vi "Image File Dialog.vi"(11 "Control Ref Queue":T2) -> ()   [LabVIEW 2020, in "3D Plot.lvclass"]
uses:
  <vilib>/Math Plots/3D Math Plots/3D Plot/3D Plot/3D Plot.lvclass
  <vilib>/Math Plots/3D Math Plots/3D Plot/Action String/3DMathPlot Ctrl Act Queue.ctl
  <vilib>/Math Plots/3D Math Plots/3D Plot/Action String/3DMathPlot Ctrl Act Cluster.ctl
  <vilib>/Math Plots/3D Math Plots/3D Plot/Action String/3DMathPlot State Class.ctl
panel:
  in  "Warning Message":string="File path is invalid."
  in  "Export":string="Export"
  in  "Save":string="Save"
  in  "Tab Control":enum32{"Appearance", "Input & Output"}(tab)
  in  "Help":bool
  in  "Cancel":bool
  in  "OK":bool
  in  "Path":path
  in  "To File":bool
  in  "To Clipboard":bool=TRUE
  in  "File Format":T1(radio)
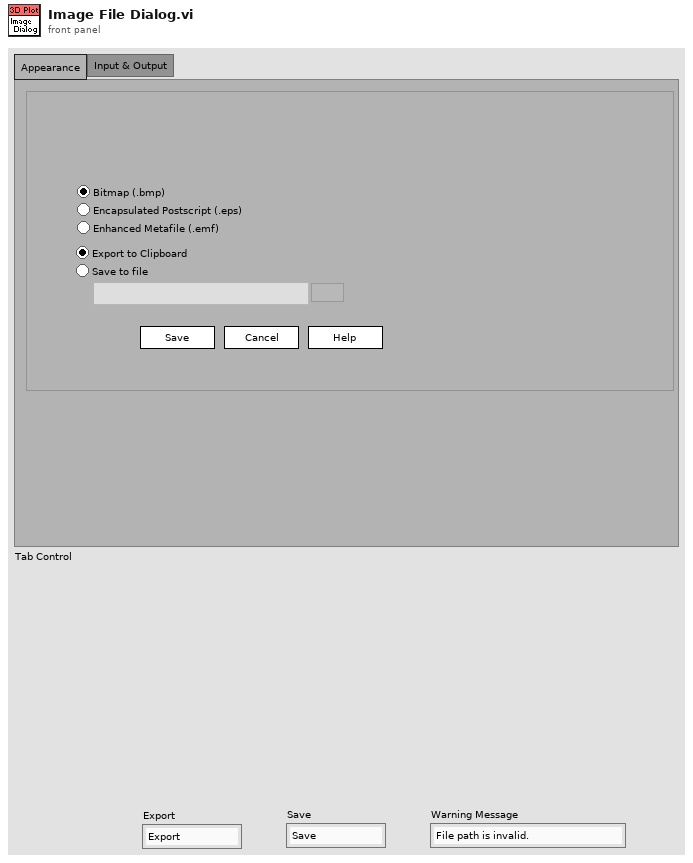
[diagram p1: front panel]
types:
  T1 = enum32{"Bitmap", "Postscript", "Metafile", "Mac PICT"}
  T2 = typedef "3DMathPlot Ctrl Act Queue.ctl" = refnum<queue>
  T3 = enum8{"Enabled", "Disabled", "Disabled and Grayed Out"}
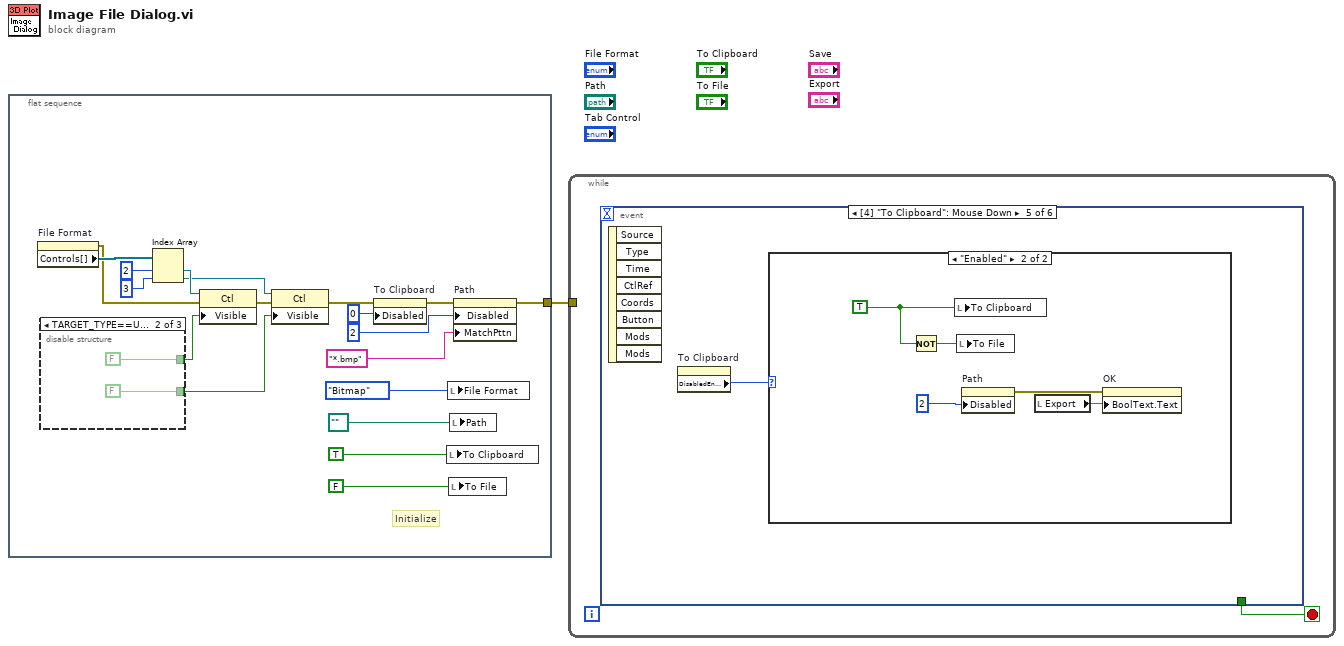
[diagram p0: block diagram]
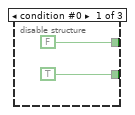
[diagram p2: hidden frame]
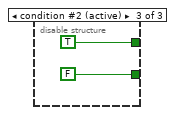
[diagram p3: hidden frame]
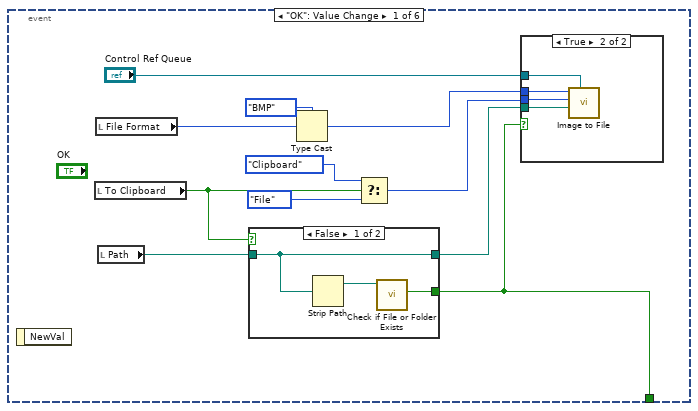
[diagram p4: hidden frame]
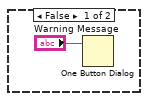
[diagram p5: hidden frame]
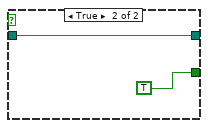
[diagram p6: hidden frame]
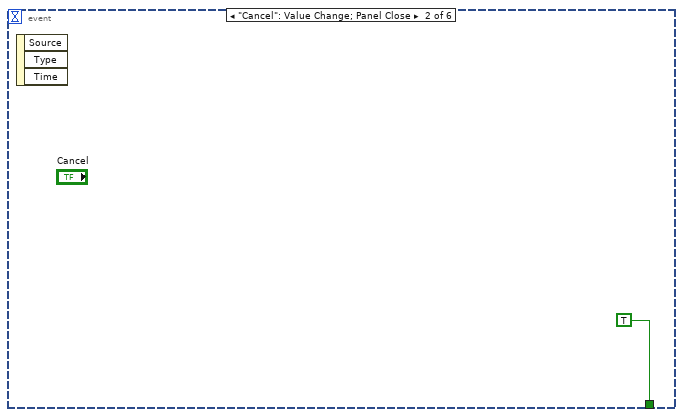
[diagram p7: hidden frame]
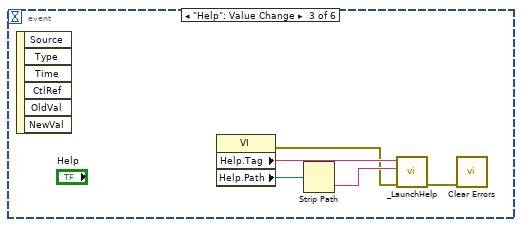
[diagram p8: hidden frame]
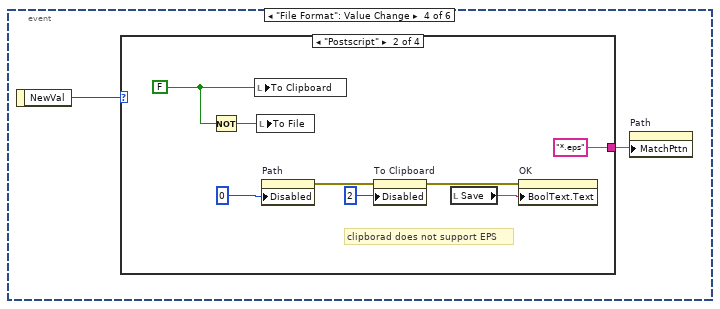
[diagram p9: hidden frame]
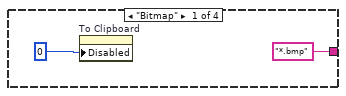
[diagram p10: hidden frame]
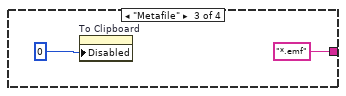
[diagram p11: hidden frame]
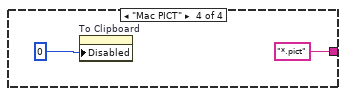
[diagram p12: hidden frame]
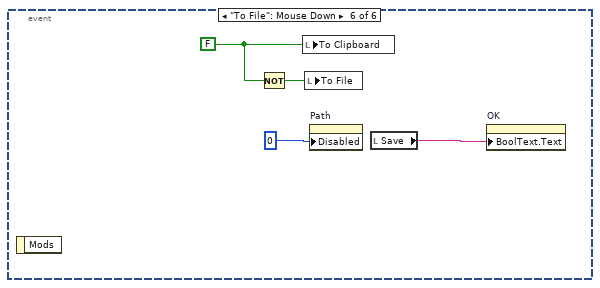
[diagram p14: hidden frame]
diagram:
  n1 = flat-sequence {
    tunnel: [w17] -> w1
    frame #0 {
      # "Initialize"
      n2 = property on="File Format" class="RadioBtnsControl (strict)"() -> (error out=w8:errorcluster, "Controls[]"=w11:refnum<vi>[])  [unwired: 2 in, 1 out]
      n3 = disable-structure shown="TARGET_TYPE==Unix" {
        disable-tunnel: [FALSE ("Visible") FALSE ("Visible") TRUE ("Visible")] -> w3
        disable-tunnel: [TRUE ("Visible") FALSE ("Visible") FALSE ("Visible")] -> w2
        frame condition #0 {
        }
        frame condition #1 {
        }
        frame condition #2 (active) {
        }
      }
      n4 = Index Array(array=w11, index #1=2 ("y"), index #2=3 ("y")) -> (element #1=w10:refnum<vi>, element #2=w6:refnum<vi>)
      n5 = property class="Ctl"(reference=w10, error in=w8, "Visible"=w3) -> (error out=w5:errorcluster)  [unwired: 1 out]
      n6 = property class="Ctl"(reference=w6, error in=w5, "Visible"=w2) -> (error out=w4:errorcluster)  [unwired: 1 out]
      n7 = property on="To Clipboard" class="Bool (strict)"(error in=w4, "Disabled"=u8 0) -> (error out=w16:errorcluster)  [unwired: 1 in, 1 out]
      n8 = local write "To Clipboard"(TRUE ("To Clipboard")) -> ()
      n9 = local write "File Format"(T1."Bitmap" ("File Format")) -> ()
      n10 = local write "To File"(FALSE ("To File")) -> ()
      n11 = local write "Path"(path "" ("Path")) -> ()
      n12 = property on="Path" class="Path"(error in=w16, "Disabled"=u8 2, "MatchPttn"="*.bmp" ("Browse Options:Match Pattern")) -> (error out=w17:errorcluster)  [unwired: 1 in, 1 out]
    }
  }
  n13 = while {
    tunnel: w1 -> [_]
    stop <- w27 stop-if-true
    n14 = event shown="[4] \"To Clipboard\": Mouse Down" {
      selector: _ -> [_ _ _ _ _ _]
      dyn-events: _ -> [_ _ _ _ _ _]
      timeout: _ -> [_ _ _ _ _ _]
      tunnel: [w28 TRUE _ _ _ _] -> w27
      event "OK": Value Change {
        n15 = event-data() -> ()  [unwired: 2 out]
        n16 = local read "To Clipboard"() -> (w31:bool)
        n17 = local read "File Format"() -> (w38:T1)
        n18 = local read "Path"() -> (w30:path)
        n19 = case shown="False" w31 {
          tunnel: w30 -> [w44 w48]
          tunnel: [w44 w48] -> w29
          tunnel: [w45 TRUE ("file or folder exists?")] -> w28
          frame False {
            n20 = Strip Path(path=w44) -> (stripped path=w46:path)  [unwired: 1 out]
            n21 = call <vilib>:"Check if File or Folder Exists.vi"("path"=w46) -> ("file or folder exists?"=w45:bool)  [unwired: 1 in, 9 out]
          }
          frame True {
          }
        }
        n22 = Type Cast(type=enum32{"BMP", "EPS", "EMF", "PICT"}."BMP" ("File Type"), x=w38) -> (*(type *) &x=w37:enum32{"BMP", "EPS", "EMF", "PICT"})
        n23 = Select(t=enum32{"File", "Clipboard"}."Clipboard" ("Target"), s=w31, f=enum32{"File", "Clipboard"}."File") -> (s? t:f=w35:enum32{"File", "Clipboard"})
        n24 = case shown="True" w28 {
          tunnel: w37 -> [_ w43]
          tunnel: w35 -> [_ w42]
          tunnel: "Control Ref Queue" -> [_ w41]
          tunnel: w29 -> [_ w40]
          frame False {
            n25 = One Button Dialog(message="Warning Message") -> ()  [unwired: 2 out]
          }
          frame True {
            n26 = call <vilib>:"Image to File.vi"("Control Ref Queue"=w41, "Path"=w40, "Target"=w42, "File Type"=w43) -> ()  [unwired: 1 in, 7 out]
          }
        }
      }
      event "Cancel": Value Change; Panel Close {
        n27 = event-data() -> ()  [unwired: 4 out]
      }
      event "Help": Value Change {
        n28 = event-data() -> ()  [unwired: 7 out]
        n29 = property class="VI"() -> (error out=w51:errorcluster, "Help.Tag"=w53:string, "Help.Path"=w54:path)  [unwired: 2 in, 1 out]
        n30 = Strip Path(path=w54) -> (name=w52:string)  [unwired: 1 out]
        n31 = call <helpdir>:"_LaunchHelp.vi"("error in (no error)"=w51, "CHM or HLP filename (lvdialog.chm)"=w52, "HTML filename"=w53) -> ("error out"=w50:errorcluster)  [unwired: 4 out]
        n32 = call <vilib>:"Clear Errors.vi"("error in (no error)"=w50) -> ()  [unwired: 5 in, 2 out]
      }
      event "File Format": Value Change {
        n33 = event-data() -> ("NewVal"=w55:T1)  [unwired: 1 out]
        n34 = case shown="\"Postscript\"" w55 {
          tunnel: ["*.bmp" ("Browse Options:Match Pattern") "*.eps" ("Browse Options:Match Pattern") "*.emf" ("Browse Options:Match Pattern") "*.pict" ("Browse Options:Match Pattern")] -> w56
          frame "Bitmap" {
            n35 = property on="To Clipboard" class="Bool (strict)"("Disabled"=u8 0) -> ()  [unwired: 2 in, 2 out]
          }
          frame "Postscript" {
            w65 = FALSE
            # "clipborad does not support EPS"
            n36 = Not(x=w65) -> (.not. x?=w66:bool)
            n37 = local write "To Clipboard"(w65) -> ()
            n38 = local write "To File"(w66) -> ()
            n39 = property on="Path" class="Path"("Disabled"=u8 0) -> (error out=w61:errorcluster)  [unwired: 2 in, 1 out]
            n40 = property on="To Clipboard" class="Bool (strict)"(error in=w61, "Disabled"=u8 2) -> (error out=w60:errorcluster)  [unwired: 1 in, 1 out]
            n41 = local read "Save"() -> (w63:string)
            n42 = property on="OK" class="Bool"(error in=w60, "BoolText.Text"=w63) -> ()  [unwired: 1 in, 2 out]
          }
          frame "Metafile" {
            n43 = property on="To Clipboard" class="Bool (strict)"("Disabled"=u8 0) -> ()  [unwired: 2 in, 2 out]
          }
          frame "Mac PICT" {
            n44 = property on="To Clipboard" class="Bool (strict)"("Disabled"=u8 0) -> ()  [unwired: 2 in, 2 out]
          }
        }
        n45 = property on="Path" class="Path"("MatchPttn"=w56) -> ()  [unwired: 2 in, 2 out]
      }
      event "To Clipboard": Mouse Down {
        n46 = event-data() -> ()  [unwired: 9 out]
        n47 = property on="To Clipboard" class="Bool (strict)"() -> ("DisabledEnum"=w71:T3)  [unwired: 2 in, 2 out]
        n48 = case shown="\"Enabled\"" w71 {
          frame Default {
          }
          frame "Enabled" {
            w75 = TRUE
            n49 = Not(x=w75) -> (.not. x?=w76:bool)
            n50 = local write "To Clipboard"(w75) -> ()
            n51 = local write "To File"(w76) -> ()
            n52 = property on="Path" class="Path"("Disabled"=u8 2) -> (error out=w72:errorcluster)  [unwired: 2 in, 1 out]
            n53 = local read "Export"() -> (w73:string)
            n54 = property on="OK" class="Bool"(error in=w72, "BoolText.Text"=w73) -> ()  [unwired: 1 in, 2 out]
          }
        }
      }
      event "To File": Mouse Down {
        w79 = FALSE
        n55 = event-data() -> ()  [unwired: 2 out]
        n56 = Not(x=w79) -> (.not. x?=w80:bool)
        n57 = local write "To Clipboard"(w79) -> ()
        n58 = local write "To File"(w80) -> ()
        n59 = property on="Path" class="Path"("Disabled"=u8 0) -> ()  [unwired: 2 in, 2 out]
        n60 = local read "Save"() -> (w77:string)
        n61 = property on="OK" class="Bool"("BoolText.Text"=w77) -> ()  [unwired: 2 in, 2 out]
      }
    }
  }
